vi "SPI API Dynamic FPGA Main.vi"() -> ()   [LabVIEW 2014]
uses:
  MCP23S17/Chip Address.ctl
  <vilib>/NI/LVFPGA Adv Session Resources/OpenByNameSubVI.vi
  <vilib>/FPGAPlugInAG/Dynamic/niLvFpga_Reset_Dynamic.vi
  <vilib>/FPGAPlugInAG/Dynamic/niLvFpga_Run_Dynamic.vi
  <vilib>/rvi/interface/common/dynamic/niFpgaEscapeDelimiterAndNull.vi
  <vilib>/Utility/error.llb/Error Cluster From Error Code.vi
  <vilib>/rvi/errors/niLvFpgaAdjustHostInterfaceError.vi
  MCP23S17/Update Mode All Pins.vi
  MCP23S17/Write Digital All Pins.vi
  <vilib>/FPGAPlugInAG/Dynamic/niLvFpga_Close_Dynamic.vi
  <vilib>/rvi/interface/nirviMethod/nirviMethod.xnode
  <vilib>/NI/LVFPGA Adv Session Resources/OpenByName.xnode
  <vilib>/rvi/interface/nirviReadWriteControl/nirviReadWriteControl.xnode
  <vilib>/rvi/interface/nirviCloseFPGA/nirviCloseFPGA.xnode
  <vilib>/NI/LVFPGA Adv Session Resources/LVFPGAAdvSessionResources.lvlib
  NiFpgaLv.dll
  <vilib>/rvi/interface/Simulation/niFpgaSimulationCallBeginRW.vi
  <vilib>/FPGAPlugInAG/Dynamic/niLvFpga_WriteFifo_Dynamic.vi
  <vilib>/rvi/errors/niLvFpgaMergeErrorWithErrorCode.vi
panel:
  in  "Value":u16 format="%016b"
  in  "Boolean":bool
  out "Array":u64[](array[numeric])
  out "SPI Command":u32 format="%.0b"
  out "Transfer Length (bits)":u8
  in  "Chip Select":u8
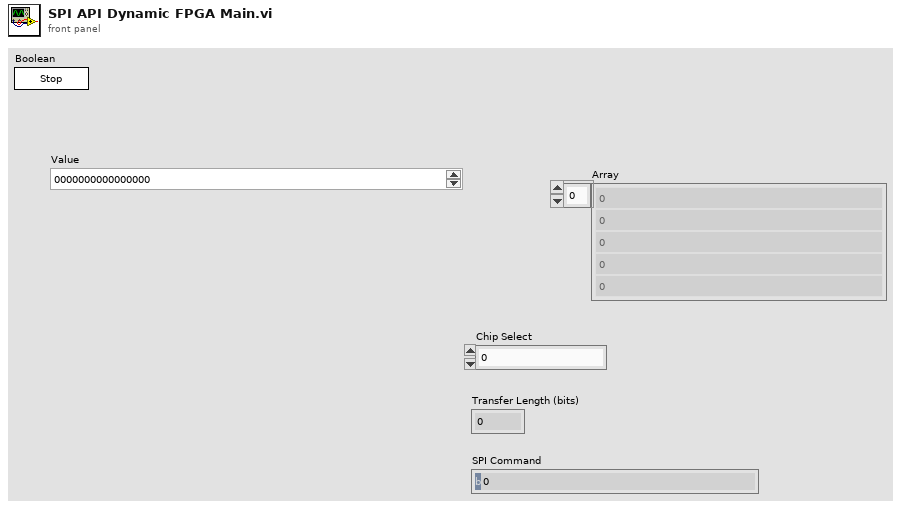
[diagram p1: front panel]
types:
  T1 = cluster{"Divide Value":u8, "Transfer Length (bits)":u8, "CS Asserted Polarity":bool, "Clock Polarity (CPOL)":bool, "Clock Phase (CPHA)":bool, "Lengthen MISO Setup":bool, "Direction Change Bit":u8, "MOSI Starts as Output":bool, "Tristatable MOSI":bool}
  T2 = typedef "Chip Address.ctl" = u8
  T3 = typedef "SPI Command.ctl" = cluster{"SPI Command":u32, "Transfer Length":u8}
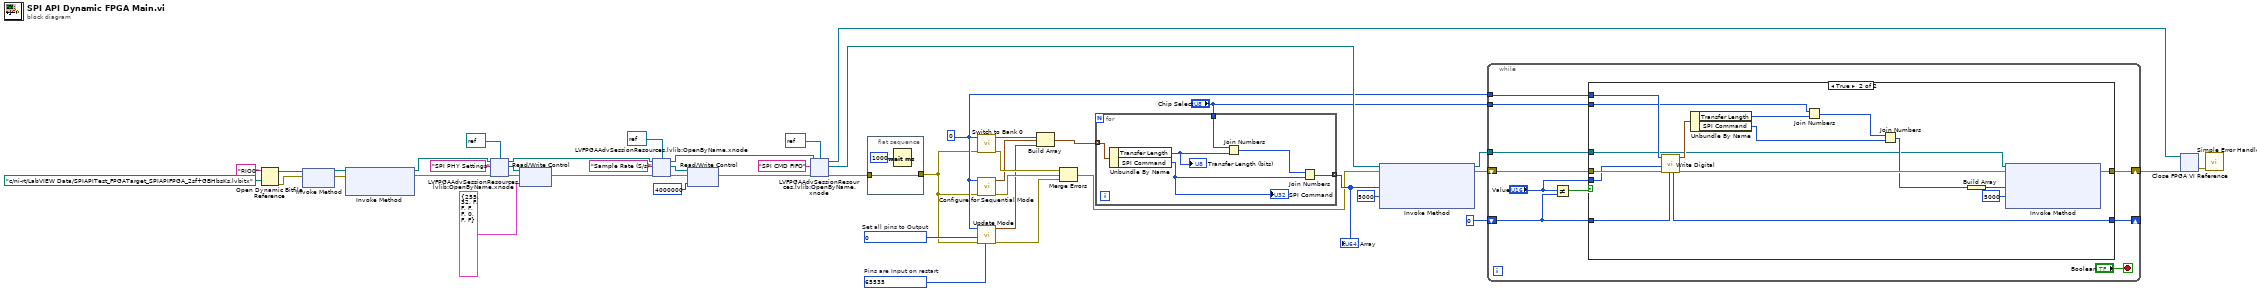
[diagram p0: block diagram]
diagram:
  w6 = T2 0 ("Chip Address (A2 A1 A0)")
  w42 = u16 0  # Set all pins to Output
  w43 = u16 65535  # Pins are Input on restart
  n1 = Open Dynamic Bitfile Reference(0:"RIO0" ("Device address"), 1:path "c:/ni-rt/LabVIEW Data/SPIAPITest_FPGATarget_SPIAPIFPGA_2sf+GBHbsKs.lvbitx" ("Bitfile path")) -> (5:w27:refnum<k20>, 8:w28:errorcluster)  [unwired: 3 in]
  n2 = xnode "Invoke Method"("FPGA VI Reference In"=w27, "error in"=w28) -> ("FPGA VI Reference Out"=w25:refnum<k20>, "error out"=w26:errorcluster)
  n3 = xnode "Invoke Method"("FPGA VI Reference In"=w25, "error in"=w26) -> ("FPGA VI Reference Out"=w23:refnum<k20>, "error out"=w22:errorcluster)  [unwired: 1 in]
  n4 = xnode "LVFPGAAdvSessionResources.lvlib:OpenByName.xnode"("FPGA VI Reference in"=w23, "Resource name in"="SPI PHY Settings", "Single resource reference type in"=refnum<k20> refnum, "Error in"=w22) -> ("Single resource reference out"=w21:refnum<k20>, "Error out"=w20:errorcluster, "FPGA VI Reference out"=w17:refnum<k20>)
  n5 = xnode "Read/Write Control"("FPGA VI Reference In"=w21, "error in"=w20, "Value"=T1 {"Divide Value"=255, "Transfer Length (bits)"=32, "CS Asserted Polarity"=FALSE, "Clock Polarity (CPOL)"=FALSE, "Clock Phase (CPHA)"=FALSE, "Lengthen MISO Setup"=FALSE, "Direction Change Bit"=0, "MOSI Starts as Output"=FALSE, "Tristatable MOSI"=FALSE} ("SPI PHY Settings")) -> ("error out"=w18:errorcluster)  [unwired: 1 out]
  n6 = xnode "LVFPGAAdvSessionResources.lvlib:OpenByName.xnode"("FPGA VI Reference in"=w17, "Resource name in"="Sample Rate (S/s)", "Single resource reference type in"=refnum<k20> refnum, "Error in"=w18) -> ("Single resource reference out"=w14:refnum<k20>, "Error out"=w15:errorcluster, "FPGA VI Reference out"=w11:refnum<k20>)
  n7 = xnode "Read/Write Control"("FPGA VI Reference In"=w14, "error in"=w15, "Value"=u32 4000000 ("Sample Rate (S/s)")) -> ("error out"=w12:errorcluster)  [unwired: 1 out]
  n8 = xnode "LVFPGAAdvSessionResources.lvlib:OpenByName.xnode"("FPGA VI Reference in"=w11, "Resource name in"="SPI CMD FIFO", "Single resource reference type in"=refnum<k20> refnum, "Error in"=w12) -> ("Single resource reference out"=w44:refnum<k20>, "Error out"=w3:errorcluster, "FPGA VI Reference out"=w29:refnum<k20>)
  n9 = flat-sequence {
    tunnel: w3 -> [w48]
    tunnel: [w48] -> w2
    frame #0 {
      n10 = Wait (ms)(milliseconds to wait=u32 1000) -> ()  [unwired: 1 out]
    }
  }
  n11 = call "Switch to Bank 0.vi"("error in (no error)"=w2, "Chip Address (A2 A1 A0)"=w6) -> ("error out"=w41:errorcluster, "SPI Command"=w38:T3)  [unwired: 8 in]
  n12 = call "Configure for Sequential Mode.vi"("error in (no error)"=w2, "Chip Address (A2 A1 A0)"=w6) -> ("error out"=w40:errorcluster, "SPI Command"=w37:T3)  [unwired: 8 in]
  n13 = call-poly "Update Mode.vi"("Mode Cache in"=w43, "error in (no error)"=w2, "Mode"=w42, "Chip Address (A2 A1 A0)"=w6) -> ("error out"=w39:errorcluster, "SPI Command"=w36:T3)  [unwired: 5 in, 1 out]
  n14 = Build Array(w38, w37, w36) -> (w35:T3[])
  n15 = Merge Errors(w41, w40, w39) -> (w32:errorcluster)
  n16 = for {
    tunnel: w35 -> [w52] mode=indexing
    tunnel: [w51] -> w34 mode=indexing
    tunnel: "Chip Select" -> [w50]
    n17 = Unbundle By Name(w52) -> ("Transfer Length"=w54:u8, "SPI Command"=w55:u32)
    "Transfer Length (bits)" <- w54
    "SPI Command" <- w55
    n18 = Join Numbers(hi=w50, lo=w54) -> ((hi.lo)=w53:u16)
    n19 = Join Numbers(hi=w53, lo=w55) -> ((hi.lo)=w51:u64)
  }
  "Array" <- w34
  n20 = xnode "Invoke Method"("FPGA VI Reference In"=w44, "error in"=w32, "Data"=w34, "Timeout (ms)"=5000) -> ("FPGA VI Reference Out"=w5:refnum<k20>, "error out"=w8:errorcluster)  [unwired: 1 out]
  n21 = while {
    shift-right: [w61] -> w7
    shift-left: w8 -> [w64]
    tunnel: w6 -> [w63]
    tunnel: w5 -> [w60]
    tunnel: "Chip Select" -> [w59]
    shift-right: [w58] -> _
    shift-left: u16 0 ("Output Cache in") -> [w57]
    stop <- "Boolean" stop-if-true
    n22 = Not Equal?(x="Value", y=w57) -> (x != y?=w62:bool)
    n23 = case shown="True" w62 {
      tunnel: w64 -> [w67 w83]
      tunnel: w63 -> [_ w82]
      tunnel: [w67 w73] -> w61
      tunnel: w60 -> [_ w72]
      tunnel: w59 -> [_ w71]
      tunnel: w57 -> [w66 w69]
      tunnel: [w66 w68] -> w58
      tunnel: "Value" -> [_ w70]
      frame False {
      }
      frame True {
        n24 = call-poly "Write Digital.vi"("Output Cache in"=w69, "error in (no error)"=w83, "Value"=w70, "Chip Address (A2 A1 A0)"=w82) -> ("error out"=w81:errorcluster, "SPI Command"=w77:T3, "Output Cache out"=w68:u16)  [unwired: 5 in]
        n25 = Unbundle By Name(w77) -> ("Transfer Length"=w79:u8, "SPI Command"=w80:u32)
        n26 = Join Numbers(hi=w71, lo=w79) -> ((hi.lo)=w78:u16)
        n27 = Join Numbers(hi=w78, lo=w80) -> ((hi.lo)=w76:u64)
        n28 = Build Array(w76) -> (w75:u64[])
        n29 = xnode "Invoke Method"("FPGA VI Reference In"=w72, "error in"=w81, "Data"=w75, "Timeout (ms)"=5000) -> ("error out"=w73:errorcluster)  [unwired: 2 out]
      }
    }
  }
  n30 = xnode "Close FPGA VI Reference"("FPGA VI Reference In"=w29, "error in"=w7) -> ("error out"=w31:errorcluster)
  n31 = call <vilib>:"Simple Error Handler.vi"("error in (no error)"=w31) -> ()  [unwired: 1 in, 8 out]
